vi "enable.vi"(8 "error in (no error)":errorcluster, 10 "model in":refnum<class "IModel.lvclass">, 11 "DefaultState in":refnum<class "DefaultState.lvclass">) -> (0 "error out":errorcluster, 2 "model out":refnum<class "IModel.lvclass">, 3 "DefaultState out":refnum<class "DefaultState.lvclass">)   [LabVIEW 2016, in "States.lvlib" / "DefaultState.lvclass"]
uses:
  DefaultState.lvclass
  IModel/IModel.lvclass
  Typedefs/CommandValue.ctl
  Typedefs/EXATypedefs.lvlib
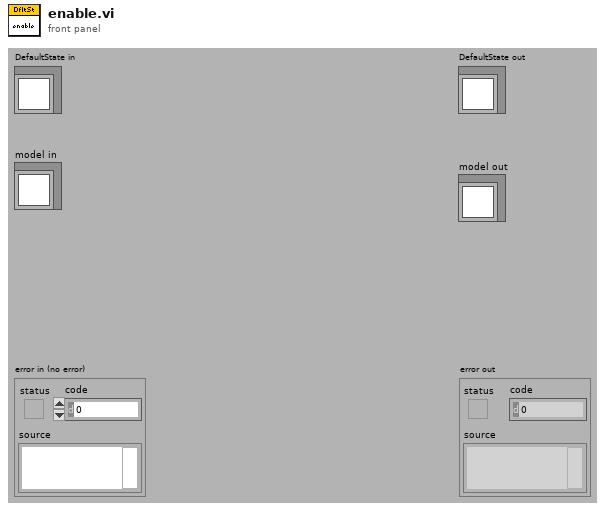
[diagram p1: front panel]
types:
  T1 = typedef "EXATypedefs.lvlib/CommandValue.ctl" = enum16{"disable", "enable", "exit", "GoToStandby", "OnHeartbeat", "OnIncomingMessagingError", "OnInterrupt", "start", "captureSpectImage", "setSpectTempSetpoint", "stopImageCapture"}
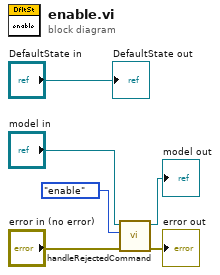
[diagram p0: block diagram]
diagram:
  n1 = call-dynamic "handleRejectedCommand.vi"("error in (no error)"="error in (no error)", "CommandValue"=CommandValue."enable", "IModel in"="model in") -> ("error out"=→"error out":errorcluster, "IModel out"=→"model out":refnum<class "IModel.lvclass">)  [unwired: 7 in]
  "DefaultState out" <- "DefaultState in"
